vi "Create X-Some Pool.vi"(6 "Parent Selection Type":enum16{"Roulette Method", "Rank Selection"}(ring), 8 "error in":errorcluster, 11 "Chromosomes In":refnum<class "IChromosome.lvclass">[](array[class])) -> (0 "error out":errorcluster, 3 "Chromosome Pool Out":refnum<class "IChromosome.lvclass">[](array[class]))   [LabVIEW 2016, in "IChromosome.lvclass"]
doc: "This VI generates a population pool from parents (solution) for mating. \nThe pool generation uses <B>Monte Carlo Method</B>:\n * Probability of selection is proportional to relative fitness\n\ni.e. For Fitness on [0,1], the member with fitness 0.75 has 75% chance of being picked.s\n\n** Stas Legedza | 06.17.2018"
uses:
  IChromosome/IChromosome.lvclass
  IChromosome/IChromosome.lvclass/IChromosome.ctl
panel:
  out "Array":dbl[](array[numeric])
  # "INPUTS"
  # "OUTPUTS"
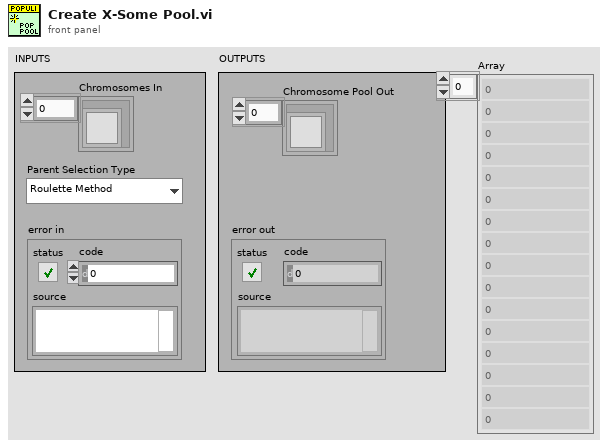
[diagram p1: front panel]
types:
  T1 = cluster{"Fitness Score":dbl, "IChromosome out":refnum<class "IChromosome.lvclass">}
  T2 = cluster{"Fitness Score":dbl, "IChromosome out":refnum<class "IChromosome.lvclass">}[]
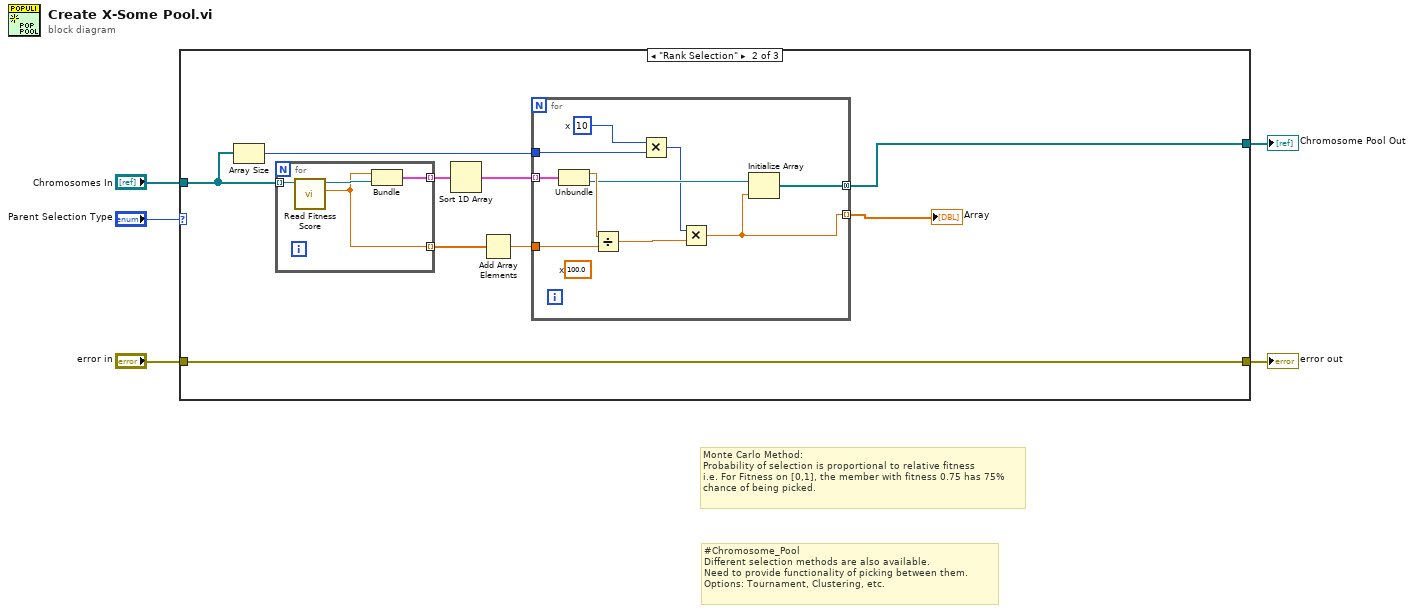
[diagram p0: block diagram]
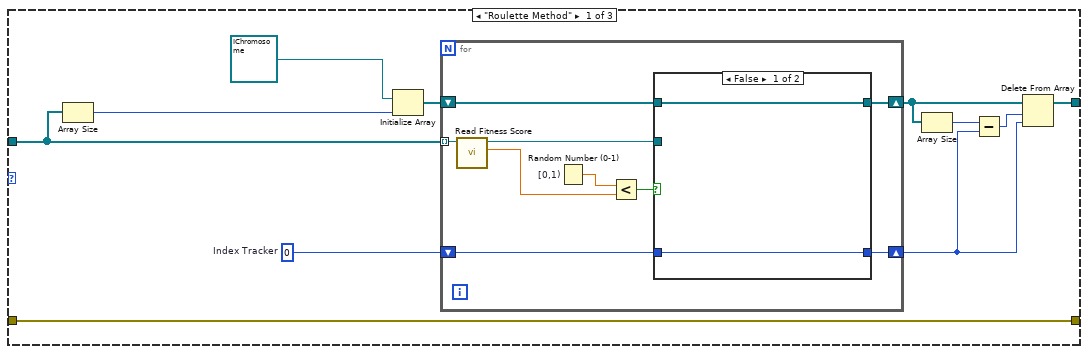
[diagram p2: hidden frame]
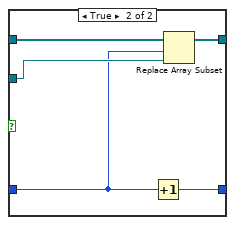
[diagram p3: hidden frame]
diagram:
  # "#Chromosome_Pool\nDifferent selection methods are also available. \nNeed to provide functionality of picking between them.\nOptions: Tournament, Clustering, etc."
  # "Monte Carlo Method:\nProbability of selection is proportional to relative fitness\ni.e. For Fitness on [0,1], the member with fitness 0.75 has 75%\nchance of being picked."
  n1 = case shown="\"Rank Selection\"" "Parent Selection Type" {
    tunnel: "Chromosomes In" -> [w13 w40 w57]
    tunnel: [w11 w34 w57] -> w4
    tunnel: "error in" -> [w6 w41 w56]
    tunnel: [w6 w41 w56] -> w1
    frame "Roulette Method" {
      w12 = 0  # Index Tracker
      n2 = Array Size(array=w13) -> (size(s)=w14:i32)
      n3 = Initialize Array(refnum<class "IChromosome.lvclass"> refnum ("Type"), w14) -> (w15:refnum<class "IChromosome.lvclass">[])
      n4 = for {
        tunnel: w13 -> [w23] mode=indexing
        shift-right: [w24] -> w10
        shift-left: w15 -> [w25]
        shift-right: [w17] -> w7
        shift-left: w12 -> [w18]
        n5 = call "Read Fitness Score.vi"("IChromosome in"=w23) -> ("Fitness Score"=w22:dbl, "IChromosome out"=w19:refnum<class "IChromosome.lvclass">)  [unwired: 8 in, 1 out]
        n6 = Random Number (0-1) "[0,1)"() -> (number: 0 to 1=w21:dbl)
        n7 = Less?(x=w21, y=w22) -> (x < y?=w20:bool)
        n8 = case shown="False" w20 {
          tunnel: w25 -> [w27 w32]
          tunnel: [w27 w31] -> w24
          tunnel: w19 -> [_ w30]
          tunnel: w18 -> [w26 w28]
          tunnel: [w26 w29] -> w17
          frame False {
          }
          frame True {
            n9 = Increment(x=w28) -> (x+1=w29:i32)
            n10 = Replace Array Subset(array=w32, new element=w30, index=w28) -> (w31:refnum<class "IChromosome.lvclass">[])
          }
        }
      }
      n11 = Array Size(array=w10) -> (size(s)=w9:i32)
      n12 = Subtract(x=w9, y=w7) -> (x-y=w8:i32)
      n13 = Delete From Array(array=w10, length=w8, index=w7) -> (array with subset deleted=w11:refnum<class "IChromosome.lvclass">[])  [unwired: 1 out]
    }
    frame "Rank Selection" {
      n14 = Array Size(array=w40) -> (size(s)=w35:i32)
      n15 = for {
        tunnel: w40 -> [w55] mode=indexing
        tunnel: [w54] -> w39 mode=indexing
        tunnel: [w52] -> w38 mode=indexing
        n16 = call "Read Fitness Score.vi"("IChromosome in"=w55) -> ("Fitness Score"=w52:dbl, "IChromosome out"=w53:refnum<class "IChromosome.lvclass">)  [unwired: 8 in, 1 out]
        n17 = Bundle("Fitness Score"=w52, "IChromosome out"=w53) -> (w54:T1)  [unwired: 1 in]
      }
      n18 = Sort 1D Array(array=w39) -> (sorted array=w37:T2)
      n19 = Add Array Elements(numeric array=w38) -> (sum=w36:dbl)
      n20 = for {
        tunnel: w37 -> [w51] mode=indexing
        tunnel: w36 -> [w49]
        tunnel: w35 -> [w45]
        tunnel: [w47] -> w34 mode=concatenating
        tunnel: [w42] -> w33 mode=indexing
        w44 = 10  # x
        (unwired) 100.0  # x
        n21 = Unbundle(w51) -> ("Fitness Score"=w50:dbl, "IChromosome out"=w48:refnum<class "IChromosome.lvclass">)
        n22 = Divide(x=w50, y=w49) -> (x/y=w46:dbl)
        n23 = Multiply(x=w44, y=w45) -> (x*y=w43:i32)
        n24 = Multiply(x=w43, y=w46) -> (x*y=w42:dbl)
        n25 = Initialize Array(w48, w42) -> (w47:refnum<class "IChromosome.lvclass">[])
      }
      "Array" <- w33
    }
    frame Default {
    }
  }
  "Chromosome Pool Out" <- w4
  "error out" <- w1
